vi "ReaderMyRio.vi"(0 "Cluster":T1={"Fahrart"=enum."Überholen", "Geschwindigkeitsmultiplikator"=0.0, "Stop"=TRUE}) -> (2 "Stop":bool, 3 "Fahrzustand":T2, 4 "Geschwindigkeitsmultiplikator":dbl)   [LabVIEW 2016]
doc: "Entschlüsselt das Array vom Laptop in die einzelnen Elemente.\nVerwendet falls kein neuer input kommt die alten"
uses:
  Control/Fahrart.ctl
  Control/GUICluster.ctl
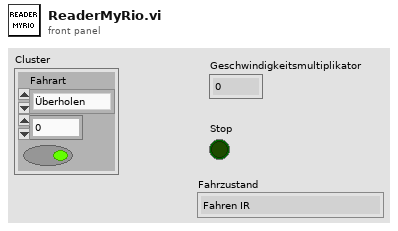
[diagram p1: front panel]
types:
  T1 = typedef "GUICluster.ctl" = cluster{"Fahrart":T2, "Geschwindigkeitsmultiplikator":dbl, "Stop":bool}
  T2 = typedef "Fahrart.ctl" = enum16{"Fahren IR", "Fahren Array", "Folgen", "Überholen"}
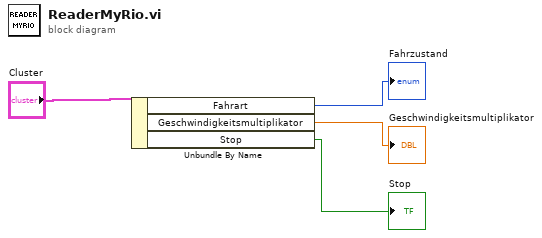
[diagram p0: block diagram]
diagram:
  n1 = Unbundle By Name("Cluster") -> ("Fahrart"=→"Fahrzustand":T2, "Geschwindigkeitsmultiplikator"=→"Geschwindigkeitsmultiplikator":dbl, "Stop"=→"Stop":bool)
